vi "Panel Origin Zero Point.vi"(8 "error in":errorcluster, 11 "VI Reference In":refnum<vi>) -> (0 "error out":errorcluster, 3 "VI Reference Out":refnum<vi>)   [LabVIEW 2018]
uses:
  <vilib>/Utility/miscctls.llb/LVPointTypeDef.ctl
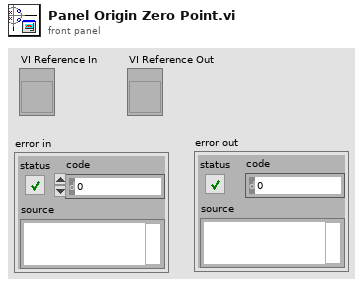
[diagram p1: front panel]
types:
  T1 = typedef "LVPointTypeDef.ctl" = cluster{"Horizontal":i16, "Vertical":i16}
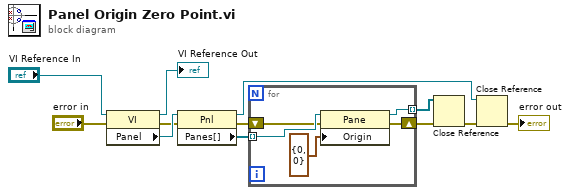
[diagram p0: block diagram]
diagram:
  n1 = property class="VI"(reference="VI Reference In", error in="error in") -> (reference out=→"VI Reference Out":refnum<vi>, error out=w5:errorcluster, "Panel"=w12:refnum<vi>)
  n2 = property class="Pnl"(reference=w12, error in=w5) -> (reference out=w6:refnum<vi>, error out=w10:errorcluster, "Panes[]"=w11:refnum<vi>[])
  n3 = for {
    tunnel: w11 -> [w17] mode=indexing
    shift-right: [w15] -> w8
    shift-left: w10 -> [w14]
    tunnel: [w13] -> w9 mode=indexing
    n4 = property class="Pane"(reference=w17, error in=w14, "Origin"=T1 {"Horizontal"=0, "Vertical"=0}) -> (reference out=w13:refnum<vi>, error out=w15:errorcluster)
  }
  n5 = Close Reference(reference=w9, error in (no error)=w8) -> (error out=w7:errorcluster)
  n6 = Close Reference(reference=w6, error in (no error)=w7) -> (error out=→"error out":errorcluster)
